vi "PFI-28000-Chan-28144_Get Coupling.vi"(8 "error in (no error)":errorcluster, 11 "PFI-28000-Chan-28144 in":refnum<class "PFI-28000-Chan-28144.lvclass">) -> (0 "error out":errorcluster, 2 "Coupling":T1, 3 "PFI-28000-Chan-28144 out":refnum<class "PFI-28000-Chan-28144.lvclass">)   [LabVIEW 2017, in "PFI-28000-Chan-28144.lvclass"]
uses:
  PFI-28000-Chan-28144.lvclass
  C:/wc/07143 Precision Filters 28000 Support/Driver/source/Channel/PFI-28000-Channel.lvclass
  PFI-28000-Chan-28144-Coupling.ctl
  Utilities/PFI-28000-Utils.lvlib
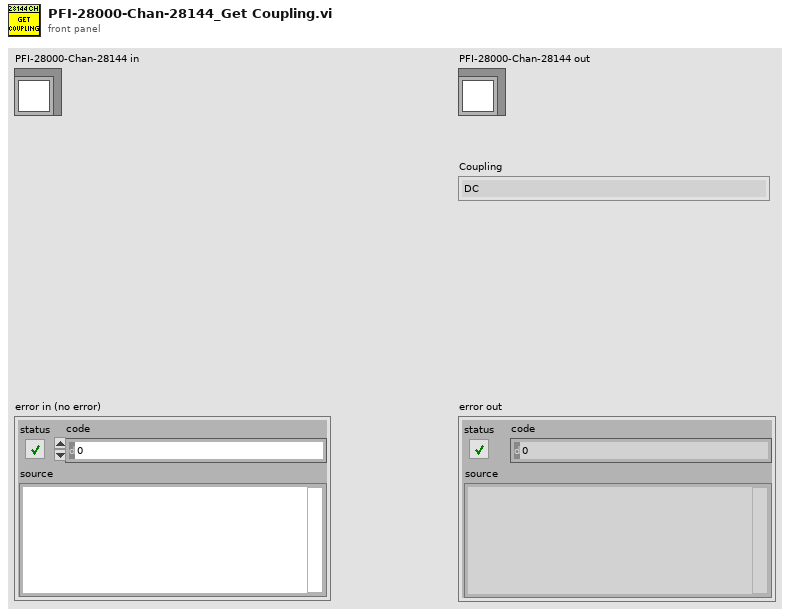
[diagram p1: front panel]
types:
  T1 = typedef "PFI-28000-Chan-28144.lvclass/PFI-28000-Chan-28144-Coupling.ctl" = enum8{"DC", "AC"}
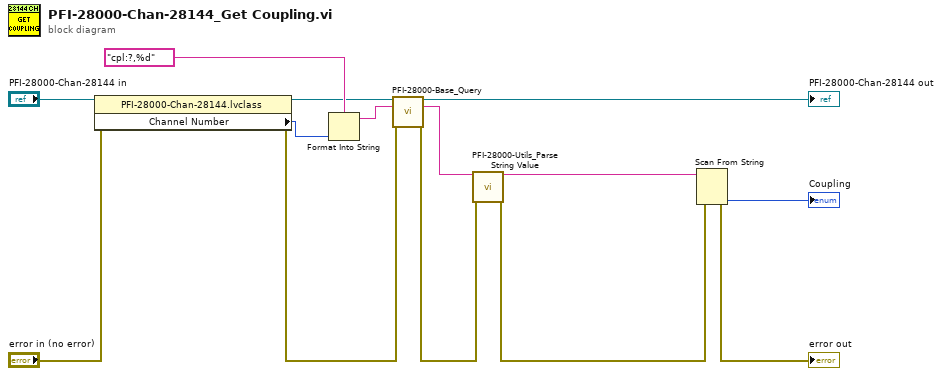
[diagram p0: block diagram]
diagram:
  n1 = property class="PFI-28000-Chan-28144.lvclass"(reference="PFI-28000-Chan-28144 in", error in="error in (no error)") -> (reference out=w8:refnum<class "PFI-28000-Chan-28144.lvclass">, error out=w6:errorcluster, "Channel Number"=w11:i32)
  n2 = Format Into String(format string="cpl:?,%d" ("empty string"), w11) -> (resulting string=w7:string)  [unwired: 2 in, 1 out]
  n3 = call-dynamic "PFI-28000-Base_Query.vi"("PFI-28000-Base in"=w8, "Command"=w7, "error in (no error)"=w6) -> ("PFI-28000-Base out"=→"PFI-28000-Chan-28144 out":refnum<class "PFI-28000-Chan-28144.lvclass">, "Response"=w4:string, "error out"=w3:errorcluster)  [unwired: 9 in, 1 out]
  n4 = call "PFI-28000-Utils_Parse String Value.vi"("String"=w4, "error in (no error)"=w3) -> ("String Value"=w1:string, "error out"=w2:errorcluster)  [unwired: 11 in, 1 out]
  n5 = Scan From String(input string=w1, error in=w2) -> (error out=→"error out":errorcluster, output 1=→"Coupling":T1)  [unwired: 3 in, 2 out]
